vi "Tracer_VIStart.vi"(10 "Calltree Offset":i32, 15 "Error In":errorcluster) -> (8 "Error Out":errorcluster)   [LabVIEW 2018, in "TracerLibrary.lvlib" / "Tracer.lvclass"]
uses:
  Tracer.lvclass
  protected/Tracer_ClassAttributes.vi
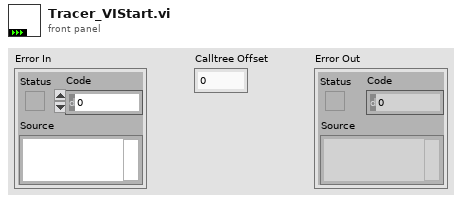
[diagram p1: front panel]
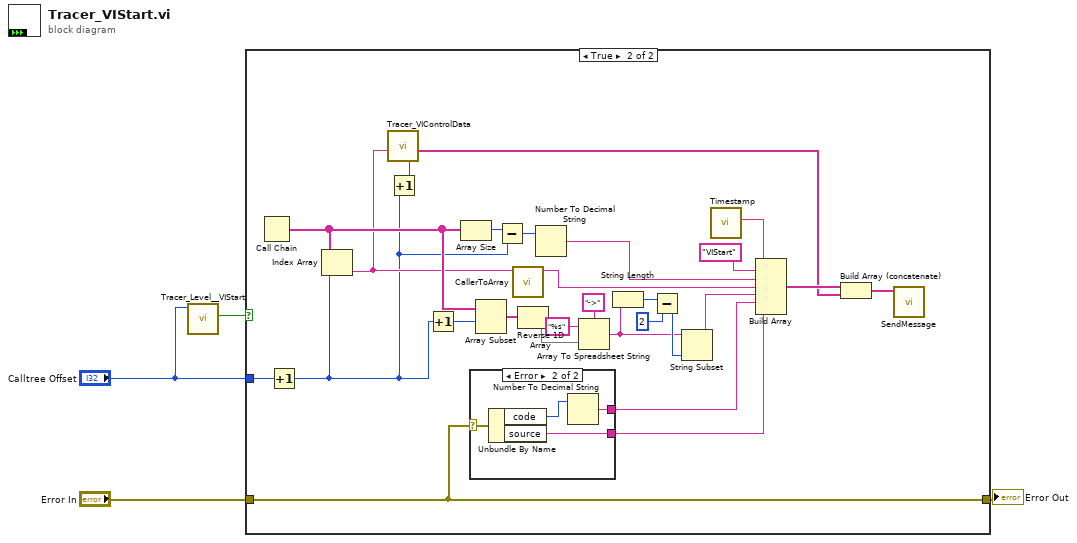
[diagram p0: block diagram]
diagram:
  n1 = call "Tracer_Level__VIStart.vi"("Calltree Level"="Calltree Offset") -> ("Trace Enabled"=w2:bool)  [unwired: 9 in, 1 out]
  n2 = case shown="True" w2 {
    tunnel: "Error In" -> [w5 w32]
    tunnel: [w5 w32] -> w3
    tunnel: "Calltree Offset" -> [_ w9]
    frame False {
    }
    frame True {
      n3 = Call Chain() -> (call chain=w14:string[])
      n4 = Increment(x=w9) -> (x+1=w6:i32)
      n5 = Index Array(array=w14, index=w6) -> (element=w11:string)
      n6 = Increment(x=w6) -> (x+1=w7:i32)
      n7 = call "Tracer_VIControlData.vi"("Calltree Level"=w7, "VI Name"=w11) -> ("Values"=w13:string[])  [unwired: 8 in, 1 out]
      n8 = Increment(x=w6) -> (x+1=w8:i32)
      n9 = Array Size(array=w14) -> (size(s)=w25:i32)
      n10 = case shown="Error" w32 {
        selector: w32 -> [_ w36]
        tunnel: [_ w34] -> w31
        tunnel: [_ w33] -> w30
        frame No Error {
        }
        frame Error {
          n11 = Unbundle By Name(w36) -> ("code"=w35:i32, "source"=w33:string)
          n12 = Number To Decimal String(number=w35) -> (decimal integer string=w34:string)  [unwired: 1 in]
        }
      }
      n13 = Array Subset(array=w14, index=w8) -> (w22:string[])  [unwired: 1 in]
      n14 = Subtract(x=w25, y=w6) -> (x-y=w24:i32)
      n15 = call "CallerToArray.vi"("String"=w11) -> ("Called"=w12:string)  [unwired: 10 in]
      n16 = Reverse 1D Array(array=w22) -> (reversed array=w21:string[])
      n17 = Number To Decimal String(number=w24) -> (decimal integer string=w23:string)  [unwired: 1 in]
      n18 = Array To Spreadsheet String(delimiter (Tab)="->", array=w21, 3:"%s" ("format string")) -> (spreadsheet string=w10:string)
      n19 = String Length(string=w10) -> (length=w17:i32)
      n20 = Subtract(x=w17, y=2) -> (x-y=w15:i32)
      n21 = String Subset(string=w10, length (rest)=w15) -> (substring=w18:string)  [unwired: 1 in]
      n22 = call "Timestamp.vi"() -> ("Date/time String"=w29:string)  [unwired: 11 in]
      n23 = Build Array(w29, "VIStart" ("element"), w23, w12, w18, w31, w30) -> (w27:string[])
      n24 = Build Array (concatenate)(w27, w13) -> (w26:string[])
      n25 = call "SendMessage.vi"("Msg"=w26) -> ()  [unwired: 11 in]
    }
  }
  "Error Out" <- w3
